vi "OddorEven.vi"(11 "Numeric":i32) -> (2 "Boolean":bool, 3 "Boolean 2":bool)   [LabVIEW 2014]
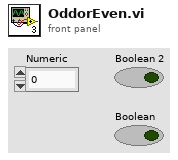
[diagram p1: front panel]
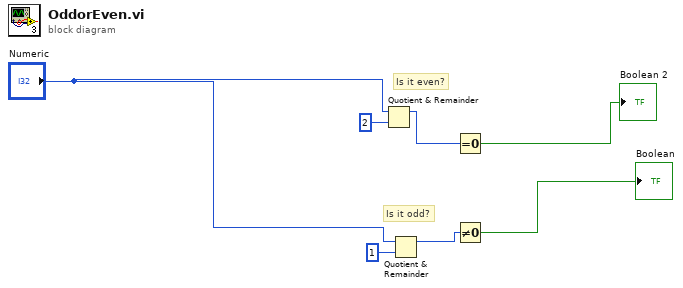
[diagram p0: block diagram]
diagram:
  # "Is it odd?"
  # "Is it even?"
  n1 = Quotient & Remainder(x="Numeric", y=2) -> (x-y*floor(x/y)=w3:i32)  [unwired: 1 out]
  n2 = Quotient & Remainder(x="Numeric", y=1) -> (x-y*floor(x/y)=w4:i32)  [unwired: 1 out]
  n3 = Equal To 0?(x=w3) -> (x = 0?=→"Boolean 2":bool)
  n4 = Not Equal To 0?(x=w4) -> (x != 0?=→"Boolean":bool)
